vi "F10.vi"(8 "error in (no error)":errorcluster) -> (0 "error out":errorcluster)   [LabVIEW 2011]
uses:
  user32.dll
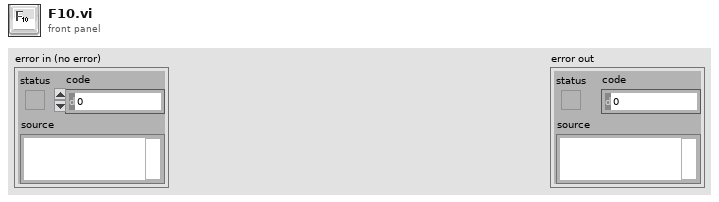
[diagram p1: front panel]
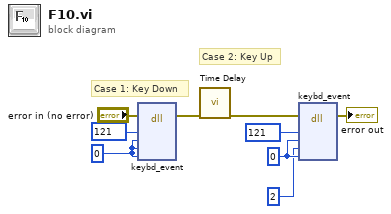
[diagram p0: block diagram]
diagram:
  w5 = u8 0 ("bScan")
  w8 = u8 0 ("bScan")
  # "Case 1: Key Down"
  # "Case 2: Key Up"
  n1 = dll-call lib="user32.dll" fn="keybd_event"(error in="error in (no error)", "bVk"=u8 121 ("Virtual Key"), "bScan"=w5, "dwFlags"=w5, "dwExtraInfo"=w5) -> (error out=w4:errorcluster)  [unwired: 7 in, 1 out]
  n2 = call "Time Delay"("error in (no error)"=w4) -> ("error out"=w3:errorcluster)  [unwired: 10 in]
  n3 = dll-call lib="user32.dll" fn="keybd_event"(error in=w3, "bVk"=u8 121 ("Virtual Key"), "bScan"=w8, "dwFlags"=u32 2, "dwExtraInfo"=w8) -> (error out=→"error out":errorcluster)  [unwired: 7 in, 1 out]
